vi "Translator.vi"(8 "error in (no error)":errorcluster, 11 "Input":variant) -> (0 "error out":errorcluster, 3 "Output":variant)   [LabVIEW 2014, in "Arduino Rotary Encoder.lvlib" / "Encoder.lvclass"]
doc: "An example of how to create the Translator to convert the LabVIEW VIs to Arduino C code."
uses:
  Encoder.lvclass
panel:
  out "Outputs":string[](array[string])
  out "Inputs":string[](array[string])
  out "Output Datatypes":string[](array[string])
  out "Input Datatypes":string[](array[string])
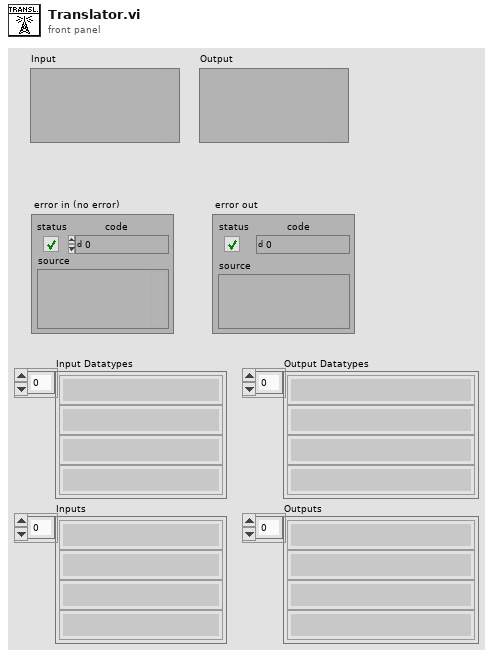
[diagram p1: front panel]
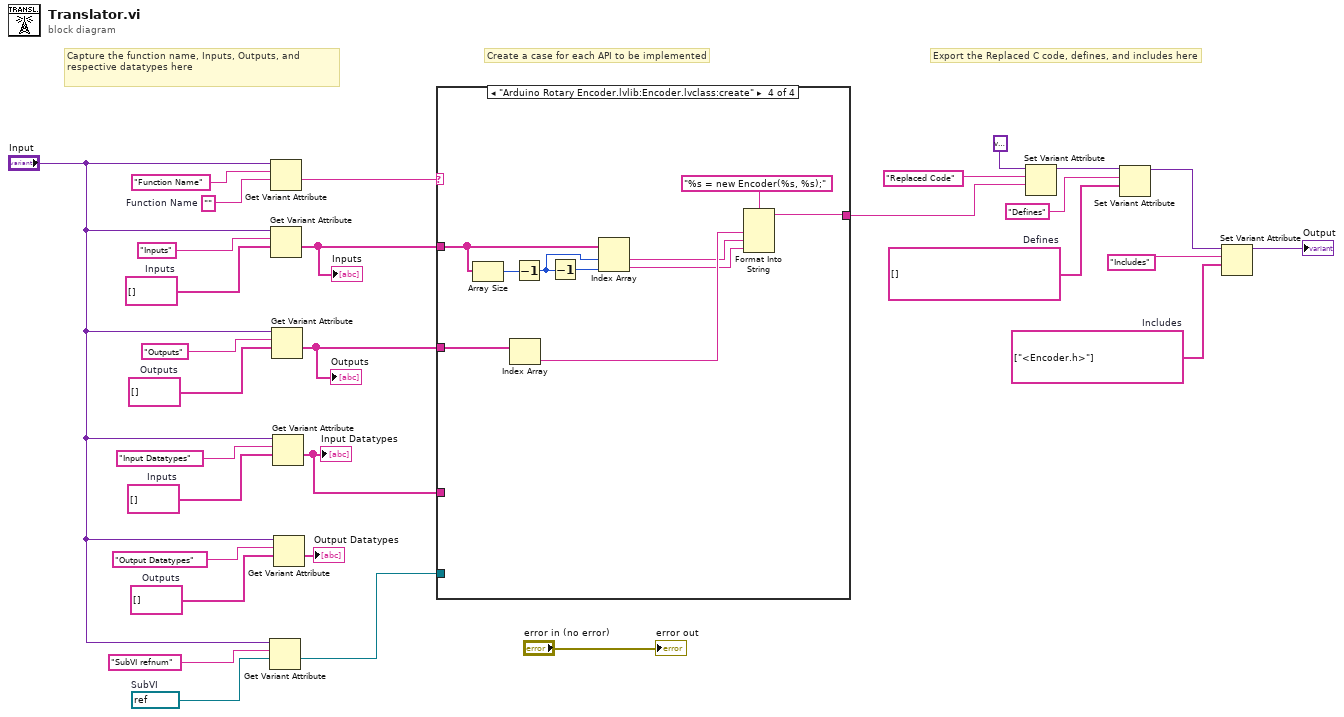
[diagram p0: block diagram]
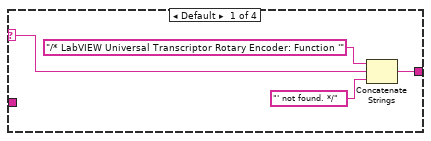
[diagram p2: hidden frame]
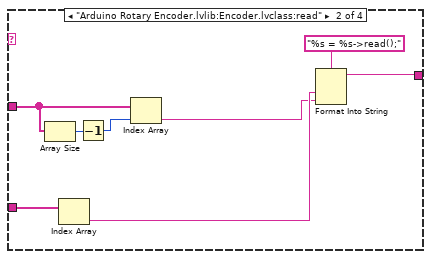
[diagram p3: hidden frame]
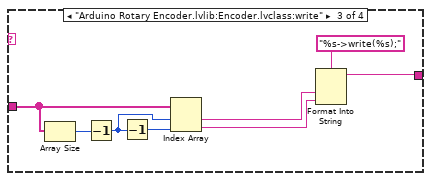
[diagram p4: hidden frame]
diagram:
  w2 = refnum<vi> refnum  # SubVI
  w6 = string[] []  # Defines
  w15 = string[] []  # Outputs
  w16 = string[] []  # Inputs
  w21 = string[] ["<Encoder.h>"]  # Includes
  w26 = string[] []  # Outputs
  w27 = string[] []  # Inputs
  w28 = ""  # Function Name
  # "Capture the function name, Inputs, Outputs, and respective datatypes here"
  # "Export the Replaced C code, defines, and includes here"
  # "Create a case for each API to be implemented"
  n1 = Get Variant Attribute(Variant="Input", name="SubVI refnum", default value (empty Variant)=w2) -> (value=w1:refnum<vi>)  [unwired: 1 in, 3 out]
  n2 = Get Variant Attribute(Variant="Input", name="Function Name", default value (empty Variant)=w28) -> (value=w23:string)  [unwired: 1 in, 3 out]
  n3 = Get Variant Attribute(Variant="Input", name="Inputs", default value (empty Variant)=w27) -> (value=w11:string[])  [unwired: 1 in, 3 out]
  "Inputs" <- w11
  n4 = Get Variant Attribute(Variant="Input", name="Outputs", default value (empty Variant)=w26) -> (value=w12:string[])  [unwired: 1 in, 3 out]
  "Outputs" <- w12
  n5 = Get Variant Attribute(Variant="Input", name="Input Datatypes", default value (empty Variant)=w16) -> (value=w5:string[])  [unwired: 1 in, 3 out]
  "Input Datatypes" <- w5
  n6 = Get Variant Attribute(Variant="Input", name="Output Datatypes", default value (empty Variant)=w15) -> (value=→"Output Datatypes":string[])  [unwired: 1 in, 3 out]
  n7 = case shown="\"Arduino Rotary Encoder.lvlib:Encoder.lvclass:create\"" w23 {
    selector: w23 -> [w33 _ _ _]
    tunnel: [w31 w41 w50 w60] -> w22
    tunnel: w11 -> [_ w38 w48 w58]
    tunnel: w12 -> [_ w42 _ w54]
    tunnel: w5 -> [_ _ _ _]
    tunnel: w1 -> [_ _ _ _]
    frame Default {
      n8 = Concatenate Strings("/* LabVIEW Universal Transcriptor Rotary Encoder: Function '", w33, "' not found. */") -> (w31:string)
    }
    frame "Arduino Rotary Encoder.lvlib:Encoder.lvclass:read" {
      n9 = Array Size(array=w38) -> (size(s)=w37:i32)
      n10 = Index Array(array=w42) -> (element=w39:string)  [unwired: 1 in]
      n11 = Decrement(x=w37) -> (x-1=w36:i32)
      n12 = Index Array(array=w38, index=w36) -> (element=w35:string)
      n13 = Format Into String(format string="%s = %s->read();", w39, w35) -> (resulting string=w41:string)  [unwired: 2 in, 1 out]
    }
    frame "Arduino Rotary Encoder.lvlib:Encoder.lvclass:write" {
      n14 = Array Size(array=w48) -> (size(s)=w47:i32)
      n15 = Decrement(x=w47) -> (x-1=w44:i32)
      n16 = Decrement(x=w44) -> (x-1=w45:i32)
      n17 = Index Array(array=w48, index #1=w44, index #2=w45) -> (element #1=w46:string, element #2=w43:string)
      n18 = Format Into String(format string="%s->write(%s);", w46, w43) -> (resulting string=w50:string)  [unwired: 2 in, 1 out]
    }
    frame "Arduino Rotary Encoder.lvlib:Encoder.lvclass:create" {
      n19 = Array Size(array=w58) -> (size(s)=w57:i32)
      n20 = Index Array(array=w54) -> (element=w53:string)  [unwired: 1 in]
      n21 = Decrement(x=w57) -> (x-1=w55:i32)
      n22 = Decrement(x=w55) -> (x-1=w56:i32)
      n23 = Index Array(array=w58, index #1=w55, index #2=w56) -> (element #1=w52:string, element #2=w51:string)
      n24 = Format Into String(format string="%s = new Encoder(%s, %s);", w53, w52, w51) -> (resulting string=w60:string)  [unwired: 2 in, 1 out]
    }
  }
  n25 = Set Variant Attribute(Variant=variant ("variant"), name="Replaced Code", value=w22) -> (Variant out=w9:variant)  [unwired: 1 in, 2 out]
  n26 = Set Variant Attribute(Variant=w9, name="Defines", value=w6) -> (Variant out=w8:variant)  [unwired: 1 in, 2 out]
  n27 = Set Variant Attribute(Variant=w8, name="Includes", value=w21) -> (Variant out=→"Output":variant)  [unwired: 1 in, 2 out]
  "error out" <- "error in (no error)"
